vi "AddCounterWithPLCSignal.vi"(6 "CycleTimeMonitorIN":T2(array[cluster]), 7 "CycleTimeArrayIN":T3(array[cluster]), 8 "Hour":string, 9 "Counters Monitor Array IN":T1(array[cluster]), 10 "MachineName":string, 11 "PLC_Bool_IN":bool) -> (0 "CycleTimeMonitorOUT":T2(array[cluster]), 1 "Counters Monitor Array OUT":T1(array[cluster]), 4 "CycleTimeArrayOUT":T3(array[cluster]))   [LabVIEW 2017]
panel:
  in  "Tab Control":enum32{"Page 1", "Page 2"}(tab)
  out "Hour:Minute:Sec":string
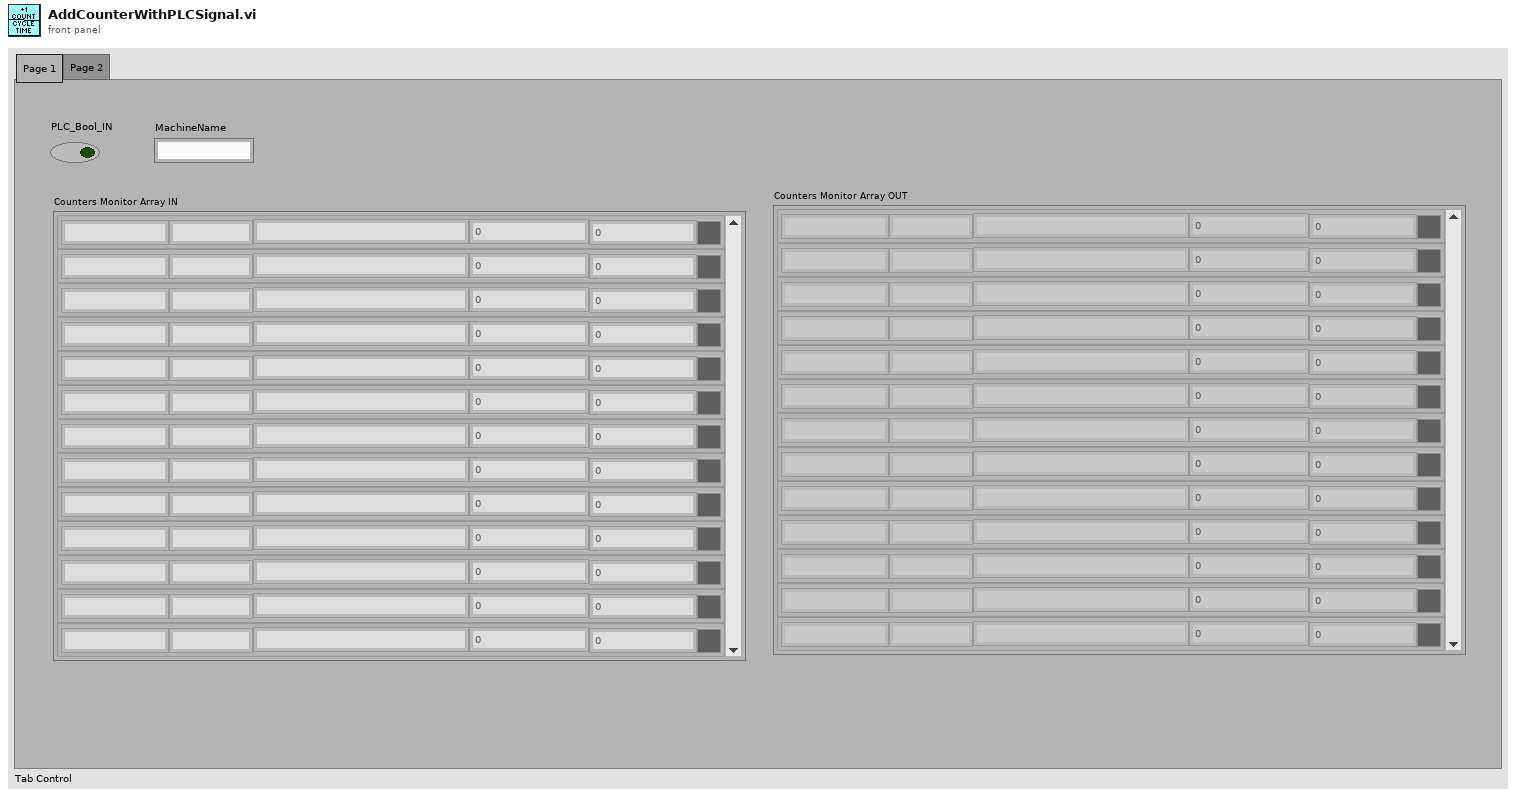
[diagram p1: front panel]
types:
  T1 = cluster{"MachineName":string, "ComponentName":string, "StoppageAlarmCounter":i32, "CurrentCount":i32, "StatusColorBox":u32, "ToolCribPartNumber":string}[]
  T2 = cluster{"Connection":bool, "MachineName":string, "CycleTime":dbl}[]
  T3 = cluster{"MachineName":string, "LastHour":string}[]
  T4 = cluster{"MachineName":string, "ComponentName":string, "StoppageAlarmCounter":i32, "CurrentCount":i32, "StatusColorBox":u32, "ToolCribPartNumber":string}
  T5 = cluster{"Connection":bool, "MachineName":string, "CycleTime":dbl}
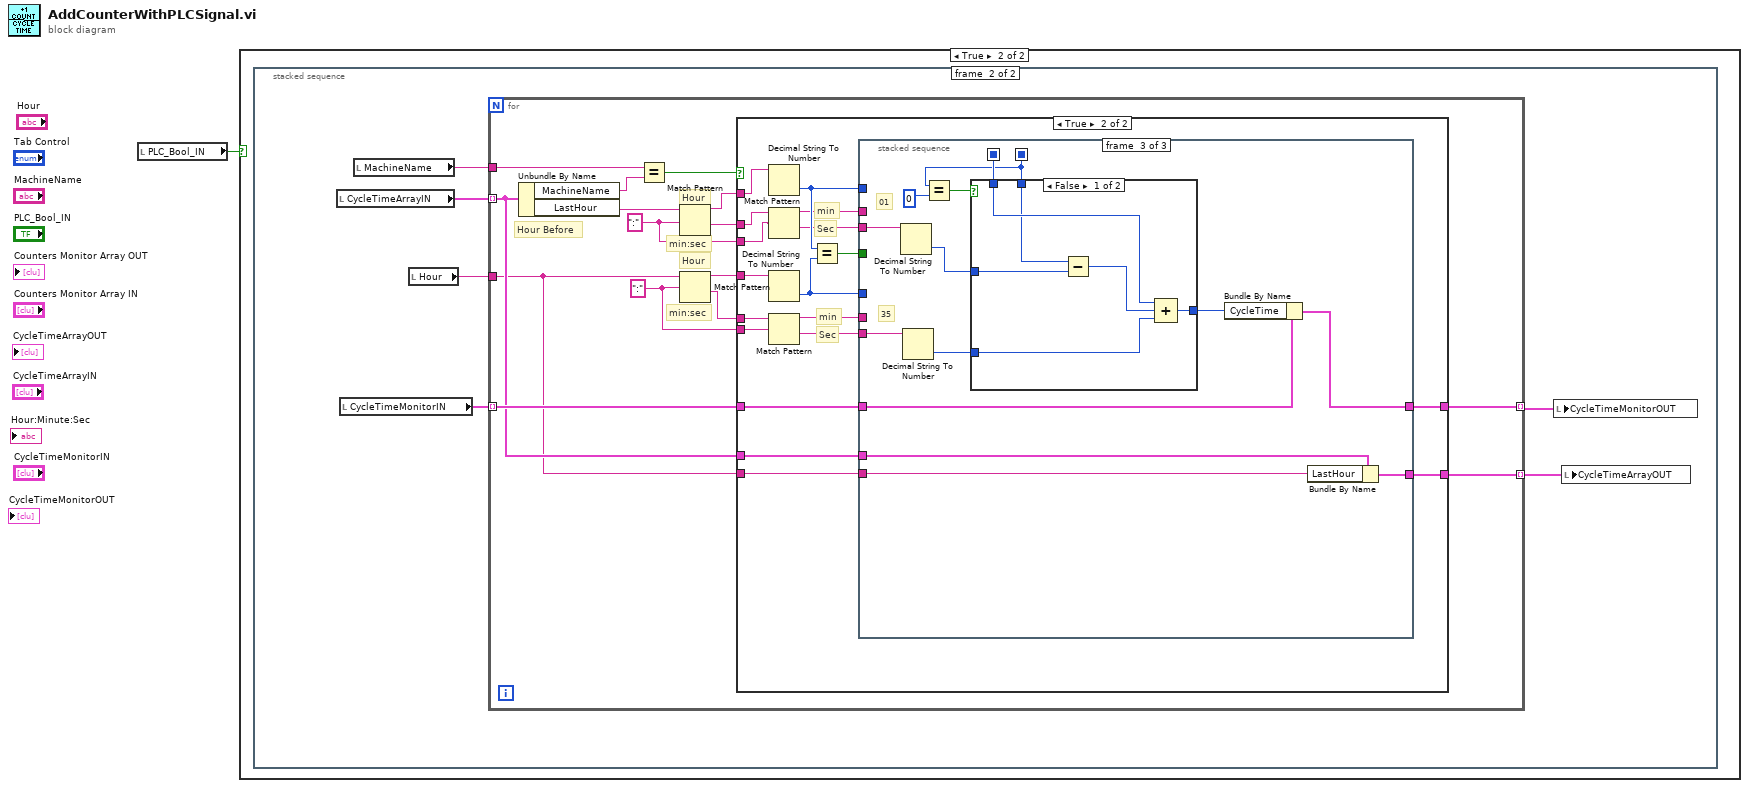
[diagram p0: block diagram]
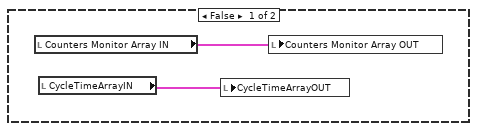
[diagram p2: hidden frame]
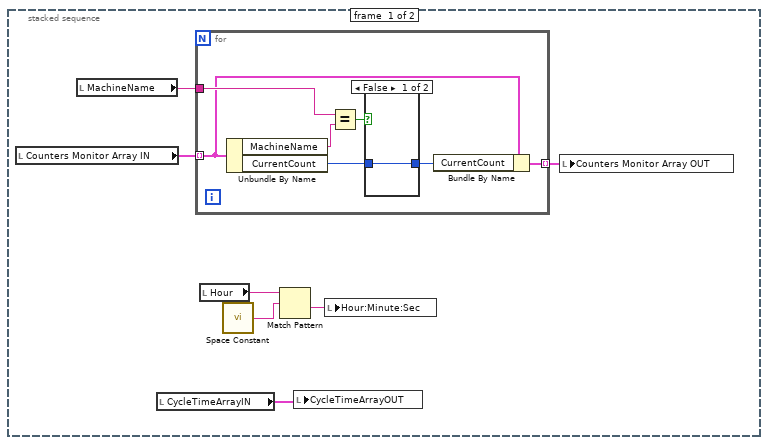
[diagram p3: hidden frame]
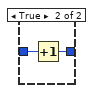
[diagram p4: hidden frame]
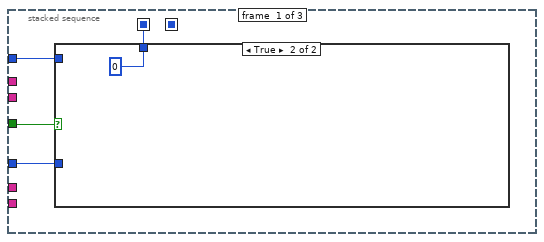
[diagram p6: hidden frame]
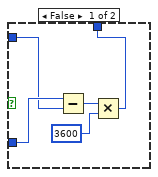
[diagram p7: hidden frame]
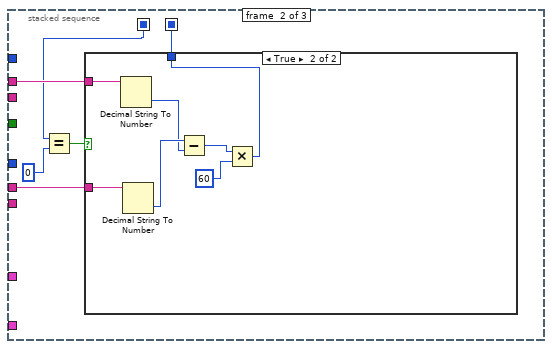
[diagram p8: hidden frame]
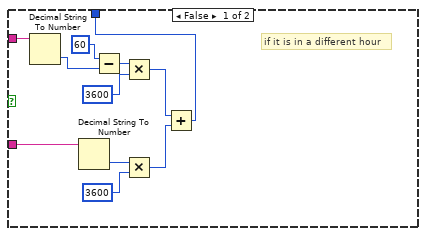
[diagram p9: hidden frame]
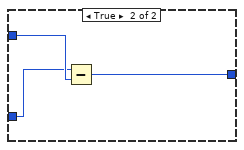
[diagram p10: hidden frame]
diagram:
  n1 = local read "PLC_Bool_IN"() -> (w1:bool)
  n2 = case shown="True" w1 {
    frame False {
      n3 = local read "Counters Monitor Array IN"() -> (w3:T1)
      n4 = local read "CycleTimeArrayIN"() -> (w2:T3)
      n5 = local write "CycleTimeArrayOUT"(w2) -> ()
      n6 = local write "Counters Monitor Array OUT"(w3) -> ()
    }
    frame True {
      n7 = stacked-sequence {
        frame #0 {
          n8 = local read "Counters Monitor Array IN"() -> (w10:T1)
          n9 = local read "MachineName"() -> (w9:string)
          n10 = local read "CycleTimeArrayIN"() -> (w4:T3)
          n11 = for {
            tunnel: w10 -> [w13] mode=indexing
            tunnel: w9 -> [w16]
            tunnel: [w11] -> w8 mode=indexing
            n12 = Unbundle By Name(w13) -> ("MachineName"=w17:string, "CurrentCount"=w14:i32)
            n13 = Equal?(x=w16, y=w17) -> (x = y?=w15:bool)
            n14 = case shown="False" w15 {
              tunnel: w14 -> [w18 w20]
              tunnel: [w18 w19] -> w12
              frame False {
              }
              frame True {
                n15 = Increment(x=w20) -> (x+1=w19:i32)
              }
            }
            n16 = Bundle By Name(cluster=w13, "CurrentCount"=w12) -> (w11:T4)
          }
          n17 = local read "Hour"() -> (w7:string)
          n18 = call <vilib>:"Space Constant.vi"() -> ("String"=w6:string)
          n19 = Match Pattern(string=w7, regular expression=w6) -> (after substring=w5:string)  [unwired: 1 in, 3 out]
          n20 = local write "CycleTimeArrayOUT"(w4) -> ()
          n21 = local write "Hour:Minute:Sec"(w5) -> ()
          n22 = local write "Counters Monitor Array OUT"(w8) -> ()
        }
        frame #1 {
          n23 = local read "CycleTimeArrayIN"() -> (w25:T3)
          n24 = local read "CycleTimeMonitorIN"() -> (w23:T2)
          n25 = local read "MachineName"() -> (w26:string)
          n26 = local read "Hour"() -> (w24:string)
          n27 = for {
            tunnel: w26 -> [w40]
            tunnel: w25 -> [w29] mode=indexing
            tunnel: w24 -> [w28]
            tunnel: w23 -> [w31] mode=indexing
            tunnel: [w30] -> w22 mode=indexing
            tunnel: [w27] -> w21 mode=indexing
            w33 = ":"
            w32 = ":"
            # "min:sec"
            # "Hour Before"
            # "Hour"
            # "min:sec"
            # "Hour"
            n28 = Unbundle By Name(w29) -> ("MachineName"=w41:string, "LastHour"=w39:string)
            n29 = Equal?(x=w40, y=w41) -> (x = y?=w38:bool)
            n30 = Match Pattern(string=w39, regular expression=w32) -> (before substring=w37:string, after substring=w35:string)  [unwired: 1 in, 2 out]
            n31 = Match Pattern(string=w28, regular expression=w33) -> (before substring=w36:string, after substring=w34:string)  [unwired: 1 in, 2 out]
            n32 = case shown="True" w38 {
              tunnel: w37 -> [_ w61]
              tunnel: w36 -> [_ w60]
              tunnel: w35 -> [_ w56]
              tunnel: w34 -> [_ w55]
              tunnel: w33 -> [_ w54]
              tunnel: w32 -> [_ w53]
              tunnel: w31 -> [w43 w48]
              tunnel: [w43 w47] -> w30
              tunnel: w29 -> [w42 w46]
              tunnel: w28 -> [_ w45]
              tunnel: [w42 w44] -> w27
              frame False {
              }
              frame True {
                # "Sec"
                # "min"
                # "Sec"
                # "min"
                n33 = Decimal String To Number(string=w61) -> (number=w57:i32)  [unwired: 2 in, 1 out]
                n34 = Match Pattern(string=w56, regular expression=w53) -> (before substring=w52:string, after substring=w51:string)  [unwired: 1 in, 2 out]
                n35 = Decimal String To Number(string=w60) -> (number=w58:i32)  [unwired: 2 in, 1 out]
                n36 = Match Pattern(string=w55, regular expression=w54) -> (before substring=w50:string, after substring=w49:string)  [unwired: 1 in, 2 out]
                n37 = Equal?(x=w57, y=w58) -> (x = y?=w59:bool)
                n38 = stacked-sequence {
                  seq-local: [w64 _ _] -> [_ w74 w107]
                  seq-local: [_ w72 _] -> [_ _ w99]
                  tunnel: w59 -> [w65 _ _]
                  tunnel: w58 -> [w63 _ _]
                  tunnel: w57 -> [w62 _ _]
                  tunnel: w52 -> [_ w77 _]
                  tunnel: w51 -> [_ _ w109]
                  tunnel: w50 -> [_ w76 _]
                  tunnel: w49 -> [_ _ w108]
                  tunnel: w48 -> [_ _ w104]
                  tunnel: [_ _ w102] -> w47
                  tunnel: w46 -> [_ _ w98]
                  tunnel: w45 -> [_ _ w97]
                  tunnel: [_ _ w96] -> w44
                  frame #0 {
                    n39 = case shown="True" w65 {
                      tunnel: [w66 0] -> w64
                      tunnel: w63 -> [w70 _]
                      tunnel: w62 -> [w69 _]
                      frame False {
                        n40 = Subtract(x=w70, y=w69) -> (x-y=w68:i32)
                        n41 = Multiply(x=w68, y=3600) -> (x*y=w66:i32)
                      }
                      frame True {
                      }
                    }
                  }
                  frame #1 {
                    n42 = Equal?(x=w74, y=0) -> (x = y?=w75:bool)
                    n43 = case shown="True" w75 {
                      tunnel: w77 -> [w88 w95]
                      tunnel: w76 -> [w87 w94]
                      tunnel: [w78 w89] -> w72
                      frame False {
                        # "if it is in a different hour"
                        n44 = Decimal String To Number(string=w88) -> (number=w82:i32)  [unwired: 2 in, 1 out]
                        n45 = Decimal String To Number(string=w87) -> (number=w84:i32)  [unwired: 2 in, 1 out]
                        n46 = Subtract(x=60, y=w82) -> (x-y=w81:i32)
                        n47 = Multiply(x=w81, y=3600) -> (x*y=w80:i32)
                        n48 = Multiply(x=w84, y=3600) -> (x*y=w79:i32)
                        n49 = Add(x=w80, y=w79) -> (x+y=w78:i32)
                      }
                      frame True {
                        n50 = Decimal String To Number(string=w95) -> (number=w92:i32)  [unwired: 2 in, 1 out]
                        n51 = Decimal String To Number(string=w94) -> (number=w93:i32)  [unwired: 2 in, 1 out]
                        n52 = Subtract(x=w93, y=w92) -> (x-y=w91:i32)
                        n53 = Multiply(x=w91, y=60) -> (x*y=w89:i32)
                      }
                    }
                  }
                  frame #2 {
                    # "35"
                    # "01"
                    n54 = Decimal String To Number(string=w109) -> (number=w106:i32)  [unwired: 2 in, 1 out]
                    n55 = Decimal String To Number(string=w108) -> (number=w105:i32)  [unwired: 2 in, 1 out]
                    n56 = Equal?(x=w99, y=0) -> (x = y?=w101:bool)
                    n57 = case shown="False" w101 {
                      tunnel: w99 -> [w111 _]
                      tunnel: w107 -> [w115 _]
                      tunnel: w106 -> [w114 w118]
                      tunnel: w105 -> [w112 w117]
                      tunnel: [w110 w116] -> w103
                      frame False {
                        n58 = Subtract(x=w111, y=w114) -> (x-y=w113:i32)
                        n59 = Compound Arithmetic op=ADD(w115, w113, w112) -> (w110:i32)
                      }
                      frame True {
                        n60 = Subtract(x=w117, y=w118) -> (x-y=w116:i32)
                      }
                    }
                    n61 = Bundle By Name(cluster=w104, "CycleTime"=w103) -> (w102:T5)
                    n62 = Bundle By Name(cluster=w98, "LastHour"=w97) -> (w96:cluster{"MachineName":string, "LastHour":string})
                  }
                }
              }
            }
          }
          n63 = local write "CycleTimeMonitorOUT"(w22) -> ()
          n64 = local write "CycleTimeArrayOUT"(w21) -> ()
        }
      }
    }
  }
